vi "ProdaNG.Units.Get.vi"(8 "error in (no error)":errorcluster, 11 "dbHandleIn":i32) -> (0 "error out":errorcluster, 1 "units simple":T1[](array[typedef]), 2 "units":T2[](array[typedef]), 3 "dbHandle":i32)   [LabVIEW 2016]
doc: "This function returns a product structure for a product, which is identified by a part and a serial number.\nImportant information: The field 'individual' was taken over from the field 'allgemein' of the legacy data directly. Because of this most products have the value 0 further on and only a few the value 1. \nParameter:\nhandle is an Integer, which is returned by the function Login() at the creation of a new connection.\nwabcoPartId is the Id of the part.\nserialNumber is the serial number of the product for the part above.\nproduct is a pointer on a product structure, which is filled if the returncode is 0. The structure must be defined in the calling program.\n\nReturncodes:\n0 No error\n< 0 ORACLE Error code\n6 (ERROR_INVALID_HANDLE) in case of an invalid handle\n1403 Record does not exist"
uses:
  Controls/ProdaNG.Unit.ctl
  Controls/ProdaNG.UnitSimple.ctl
  Controls/ProdaNG.UnitSize.ctl
  <vilib>/Utility/importsl/GetValueByPointer/datatype.ctl
  <vilib>/Utility/importsl/GetValueByPointer/GetValueByPointer.xnode
  prodllNG.dll
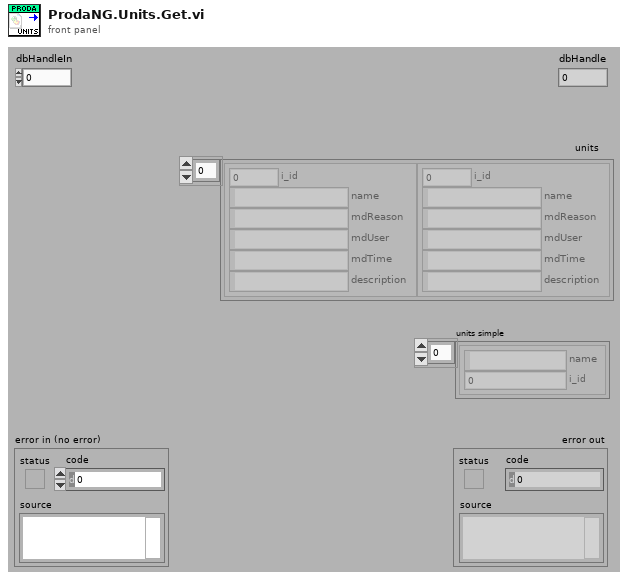
[diagram p1: front panel]
types:
  T1 = typedef "ProdaNG.UnitSimple.ctl" = cluster{"name":string, "i_id":i32}
  T2 = typedef "ProdaNG.Unit.ctl" = cluster{"i_id":i32, "name":string, "mdReason":string, "mdUser":string, "mdTime":string, "description":string}
  T3 = typedef "ProdaNG.UnitSize.ctl" = cluster{"i_id":i32, "name":i32, "mdReason":i32, "mdUser":i32, "mdTime":i32, "description":i32}
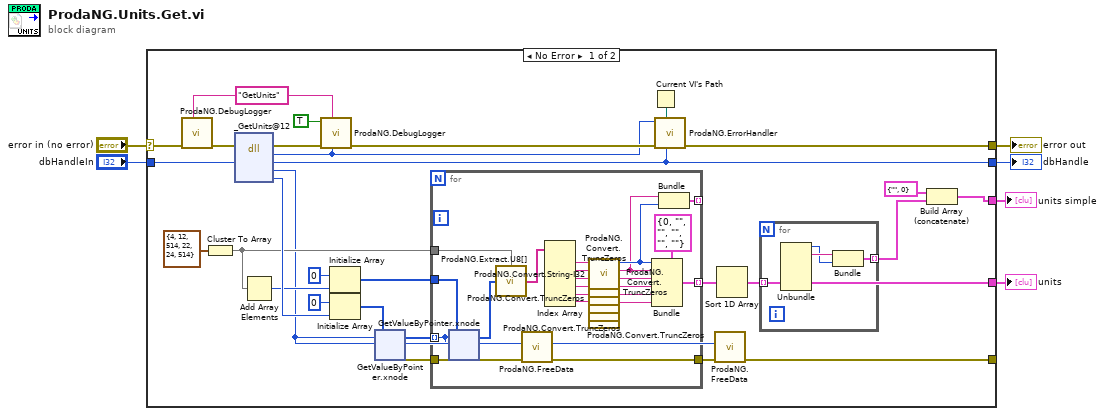
[diagram p0: block diagram]
diagram:
  n1 = case shown="No Error" "error in (no error)" {
    selector: "error in (no error)" -> [w30 w94]
    tunnel: [w35 w94] -> w5
    tunnel: "dbHandleIn" -> [w32 w93]
    tunnel: [w33 w93] -> w3
    tunnel: [w8 _] -> w2
    tunnel: [w12 _] -> _
    tunnel: [w10 _] -> w1
    frame No Error {
      w26 = "GetUnits" ("cmd")
      n2 = call "ProdaNG.DebugLogger.vi"("cmd"=w26, "error in (no error)"=w30) -> ("error out"=w29:errorcluster)  [unwired: 9 in]
      n3 = Cluster To Array(cluster=T3 {"i_id"=4, "name"=12, "mdReason"=514, "mdUser"=22, "mdTime"=24, "description"=514} ("UnitSize")) -> (array=w16:i32[])
      n4 = dll-call lib="D:/Maszup/WABCO/SVN/LineTraceSystem/SOFTWARE/sources/Database/ProdaNG/prodllNG.dll" fn="_GetUnits@12" ("ProDLL wrapper.dll:ProDLL_wrapper_GetWabcoParts_GetData")(error in=w29, "dbHandle"=w32) -> (error out=w28:errorcluster, "return type"=w25:i32, "dbHandle"=w33:i32, "units"=w11:u32, "countPtr"=w20:i32)  [unwired: 4 in, 1 out]
      n5 = Add Array Elements(numeric array=w16) -> (sum=w17:i32)
      n6 = call "ProdaNG.DebugLogger.vi"("return type"=w25, "cmd"=w26, "error in (no error)"=w28, "done? (F)"=TRUE) -> ("error out"=w27:errorcluster)  [unwired: 7 in]
      n7 = Initialize Array(u8 0 ("element"), w17) -> (w18:u8[])
      n8 = Initialize Array(u32 0 ("element"), w20) -> (w24:u32[])
      n9 = xnode "GetValueByPointer.xnode"("Pointer"=w11, "InputType"=w24) -> ("Output"=w21:u32[], "ErrorOut"=w22:errorcluster)  [unwired: 2 in]
      n10 = for {
        tunnel: w22 -> [w62]
        tunnel: w21 -> [w43] mode=indexing
        tunnel: w18 -> [w61]
        tunnel: w16 -> [w56]
        tunnel: [w55] -> w15 mode=indexing
        tunnel: [w44] -> w13
        tunnel: [w42] -> _ mode=indexing
        n11 = xnode "GetValueByPointer.xnode"("Pointer"=w43, "InputType"=w61, "ErrorIn"=w62) -> ("Output"=w58:u8[], "ErrorOut"=w45:errorcluster)  [unwired: 1 in]
        n12 = call "ProdaNG.Extract.U8[].vi"("unsigned byte array"=w58, "Sizes"=w56) -> ("Elements"=w57:string[])
        n13 = call "ProdaNG.FreeData.vi"("error in (no error)"=w45, "Pointers"=w43) -> ("error out"=w44:errorcluster)  [unwired: 9 in]
        n14 = Index Array(array=w57) -> (element #1=w59:string, element #2=w54:string, element #3=w53:string, element #4=w48:string, element #5=w47:string, element #6=w46:string)  [unwired: 6 in]
        n15 = call "ProdaNG.Convert.String-I32.vi"("unsigned byte string"=w59) -> ("32bit integer"=w41:i32)  [unwired: 10 in]
        n16 = call "ProdaNG.Convert.TruncZeros.vi"("string with \\0s"=w54) -> ("LV string"=w40:string)  [unwired: 10 in]
        n17 = call "ProdaNG.Convert.TruncZeros.vi"("string with \\0s"=w53) -> ("LV string"=w52:string)  [unwired: 10 in]
        n18 = call "ProdaNG.Convert.TruncZeros.vi"("string with \\0s"=w48) -> ("LV string"=w51:string)  [unwired: 10 in]
        n19 = call "ProdaNG.Convert.TruncZeros.vi"("string with \\0s"=w47) -> ("LV string"=w50:string)  [unwired: 10 in]
        n20 = call "ProdaNG.Convert.TruncZeros.vi"("string with \\0s"=w46) -> ("LV string"=w49:string)  [unwired: 10 in]
        n21 = Bundle(cluster=T2 {"i_id"=0, "name"="", "mdReason"="", "mdUser"="", "mdTime"="", "description"=""} ("Language"), "i_id"=w41, "name"=w40, "mdReason"=w52, "mdUser"=w51, "mdTime"=w50, "description"=w49) -> (w55:T2)
        n22 = Bundle("LV string"=w40, "32bit integer"=w41) -> (w42:cluster{"LV string":string, "32bit integer":i32})  [unwired: 1 in]
      }
      n23 = Current VI's Path() -> (path=w34:path)
      n24 = call "ProdaNG.ErrorHandler.vi"("dbHandleIn"=w33, "Path"=w34, "error in"=w27, "output_parameter"=w25) -> ("error out"=w35:errorcluster)  [unwired: 7 in]
      n25 = call "ProdaNG.FreeData.vi"("error in (no error)"=w13, "Pointers"=w11) -> ("error out"=w12:errorcluster)  [unwired: 9 in]
      n26 = Sort 1D Array(array=w15) -> (sorted array=w8:T2[])
      n27 = for {
        tunnel: w8 -> [w39] mode=indexing
        tunnel: [w36] -> w7 mode=indexing
        n28 = Unbundle(w39) -> ("i_id"=w37:i32, "name"=w38:string)  [unwired: 4 out]
        n29 = Bundle("name"=w38, "i_id"=w37) -> (w36:cluster{"name":string, "i_id":i32})  [unwired: 1 in]
      }
      n30 = Build Array (concatenate)(cluster{"LV string":string, "32bit integer":i32} {"LV string"="", "32bit integer"=0} ("cluster"), w7) -> (w10:cluster{"name":string, "i_id":i32}[])
    }
    frame Error {
    }
  }
  "error out" <- w5
  "dbHandle" <- w3
  "units" <- w2
  "units simple" <- w1
